vi "Operation (SubVI).vi"(8 "error in (no error)":errorcluster, 9 "On/Off":bool=TRUE, 10 "Operation":u16(ring) items=["Init", "0 ohm", "6 ohm", "13.2 ohm", "15 ohm", "25.9 ohm", "33 ohm", "Down", "Up", "Venable", "Firmware", "PowerSuply"], 11 "DAQmx Device Name":tag) -> (0 "error out":errorcluster)   [LabVIEW 2017]
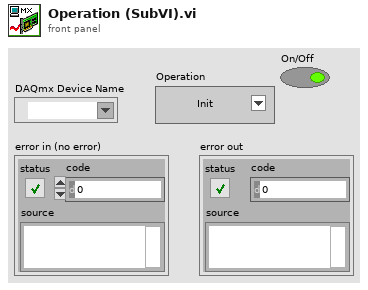
[diagram p1: front panel]
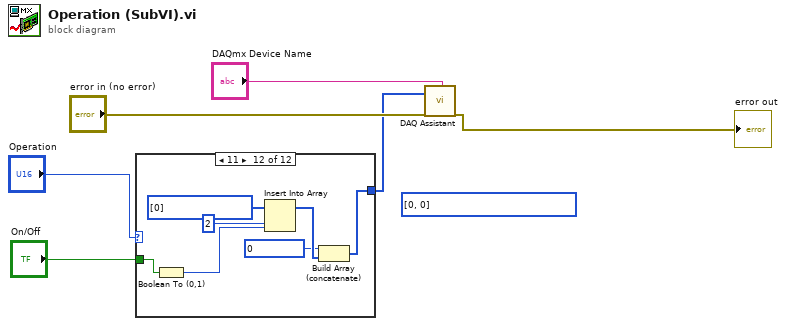
[diagram p0: block diagram]
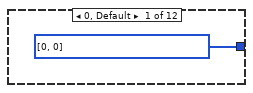
[diagram p2: hidden frame]
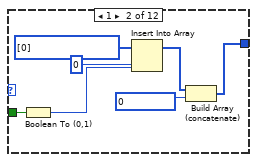
[diagram p3: hidden frame]
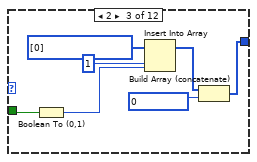
[diagram p4: hidden frame]
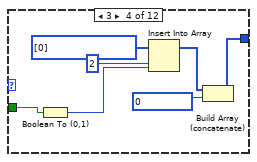
[diagram p5: hidden frame]
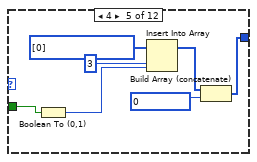
[diagram p6: hidden frame]
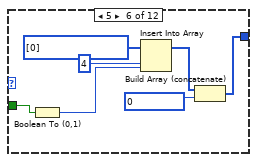
[diagram p7: hidden frame]
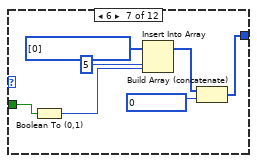
[diagram p8: hidden frame]
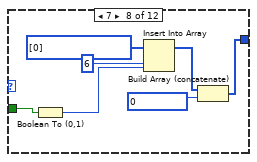
[diagram p9: hidden frame]
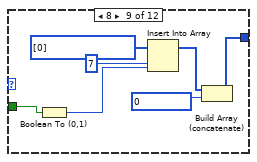
[diagram p10: hidden frame]
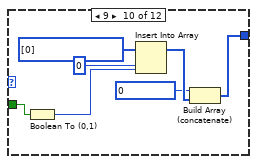
[diagram p11: hidden frame]
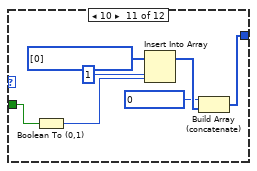
[diagram p12: hidden frame]
diagram:
  (unwired) u32[] [0, 0] ("data")
  n1 = case shown="11" "Operation" {
    tunnel: [u32[] [0, 0] ("data") w8 w15 w22 w30 w37 w44 w51 w58 w65 w72 w79] -> w2
    tunnel: "On/Off" -> [_ w12 w16 w23 w29 w36 w43 w50 w57 w64 w71 w78]
    frame 0, Default {
    }
    frame 1 {
      n2 = Boolean To (0,1)(Boolean=w12) -> (0, 1=w10:i16)
      n3 = Insert Into Array(array=u32[] [0], index=0, new element=w10) -> (w9:u32[])
      n4 = Build Array (concatenate)(w9, u32 0 ("Waveform")) -> (w8:u32[])
    }
    frame 2 {
      n5 = Boolean To (0,1)(Boolean=w16) -> (0, 1=w18:i16)
      n6 = Insert Into Array(array=u32[] [0], index=1, new element=w18) -> (w17:u32[])
      n7 = Build Array (concatenate)(w17, u32 0 ("Waveform")) -> (w15:u32[])
    }
    frame 3 {
      n8 = Boolean To (0,1)(Boolean=w23) -> (0, 1=w25:i16)
      n9 = Insert Into Array(array=u32[] [0], index=2, new element=w25) -> (w24:u32[])
      n10 = Build Array (concatenate)(w24, u32 0 ("Waveform")) -> (w22:u32[])
    }
    frame 4 {
      n11 = Boolean To (0,1)(Boolean=w29) -> (0, 1=w32:i16)
      n12 = Insert Into Array(array=u32[] [0], index=3, new element=w32) -> (w31:u32[])
      n13 = Build Array (concatenate)(w31, u32 0 ("Waveform")) -> (w30:u32[])
    }
    frame 5 {
      n14 = Boolean To (0,1)(Boolean=w36) -> (0, 1=w39:i16)
      n15 = Insert Into Array(array=u32[] [0], index=4, new element=w39) -> (w38:u32[])
      n16 = Build Array (concatenate)(w38, u32 0 ("Waveform")) -> (w37:u32[])
    }
    frame 6 {
      n17 = Boolean To (0,1)(Boolean=w43) -> (0, 1=w46:i16)
      n18 = Insert Into Array(array=u32[] [0], index=5, new element=w46) -> (w45:u32[])
      n19 = Build Array (concatenate)(w45, u32 0 ("Waveform")) -> (w44:u32[])
    }
    frame 7 {
      n20 = Boolean To (0,1)(Boolean=w50) -> (0, 1=w53:i16)
      n21 = Insert Into Array(array=u32[] [0], index=6, new element=w53) -> (w52:u32[])
      n22 = Build Array (concatenate)(w52, u32 0 ("Waveform")) -> (w51:u32[])
    }
    frame 8 {
      n23 = Boolean To (0,1)(Boolean=w57) -> (0, 1=w60:i16)
      n24 = Insert Into Array(array=u32[] [0], index=7, new element=w60) -> (w59:u32[])
      n25 = Build Array (concatenate)(w59, u32 0 ("Waveform")) -> (w58:u32[])
    }
    frame 9 {
      n26 = Boolean To (0,1)(Boolean=w64) -> (0, 1=w68:i16)
      n27 = Insert Into Array(array=u32[] [0], index=0, new element=w68) -> (w67:u32[])
      n28 = Build Array (concatenate)(u32 0 ("Waveform"), w67) -> (w65:u32[])
    }
    frame 10 {
      n29 = Boolean To (0,1)(Boolean=w71) -> (0, 1=w75:i16)
      n30 = Insert Into Array(array=u32[] [0], index=1, new element=w75) -> (w74:u32[])
      n31 = Build Array (concatenate)(u32 0 ("Waveform"), w74) -> (w72:u32[])
    }
    frame 11 {
      n32 = Boolean To (0,1)(Boolean=w78) -> (0, 1=w82:i16)
      n33 = Insert Into Array(array=u32[] [0], index=2, new element=w82) -> (w81:u32[])
      n34 = Build Array (concatenate)(u32 0 ("Waveform"), w81) -> (w79:u32[])
    }
  }
  n35 = call "DAQ Assistant"("data"=w2, "error in"="error in (no error)", "device name"="DAQmx Device Name") -> ("error out"=→"error out":errorcluster)  [unwired: 15 in, 1 out]
